vi "OCR test bench.vi"() -> ()   [LabVIEW 2017]
uses:
  <vilib>/vision/NI_Vision_Development_Module.lvlib
  <vilib>/userdefined/High Color/IMAQdx.ctl
  <vilib>/vision/Image Controls.llb/IMAQ Image.ctl
  <vilib>/vision/Avi.llb/IMAQ AVI2 Refnum.ctl
  Controls/Refnums.ctl
  Controls/Room Dimensions.ctl
  Controls/Dimensions.ctl
  Controls/Frame Grabber Data.ctl
  <vilib>/Utility/miscctls.llb/LVOutOfRangeActionTypeDef.ctl
  Controls/Crop Type.ctl
  Controls/Crop Video State.ctl
  <vilib>/vision/OCR.llb/IMAQ OCR Character Report 2.ctl
panel:
  out "Character Reports":T1[](array[typedef]) {"Character Statistics"."Threshold Range"."Upper value" format="%.2f"; "Character Statistics"."Threshold Range"."Lower value" format="%.2f"}
  in  "Range":cluster{"Lower value":sgl, "Upper value":sgl}={"Lower value"=128.0, "Upper value"=255.0} {"Upper value" format="%.2f"; "Lower value" format="%.2f"}
  out "Cropped":T2(plugin-control)
  in  "Stop Button":bool
  in  "Blue or Luminance":cluster{"Min":i32, "Max":i32}(slide)={"Min"=70, "Max"=183} scale=0.0..255.0
  in  "Green or Saturation":cluster{"Min":i32, "Max":i32}(slide)={"Min"=51, "Max"=206} scale=0.0..255.0
  in  "Red or Hue":cluster{"Min":i32, "Max":i32}(slide)={"Min"=217, "Max"=15} scale=0.0..255.0
  out "Thresh Image":T2(plugin-control)
  out "Frame":T2(plugin-control)
  out "Reference zero image":T2(plugin-control)
  in  "Frame Number":u32 max=30
  out "Read String":string
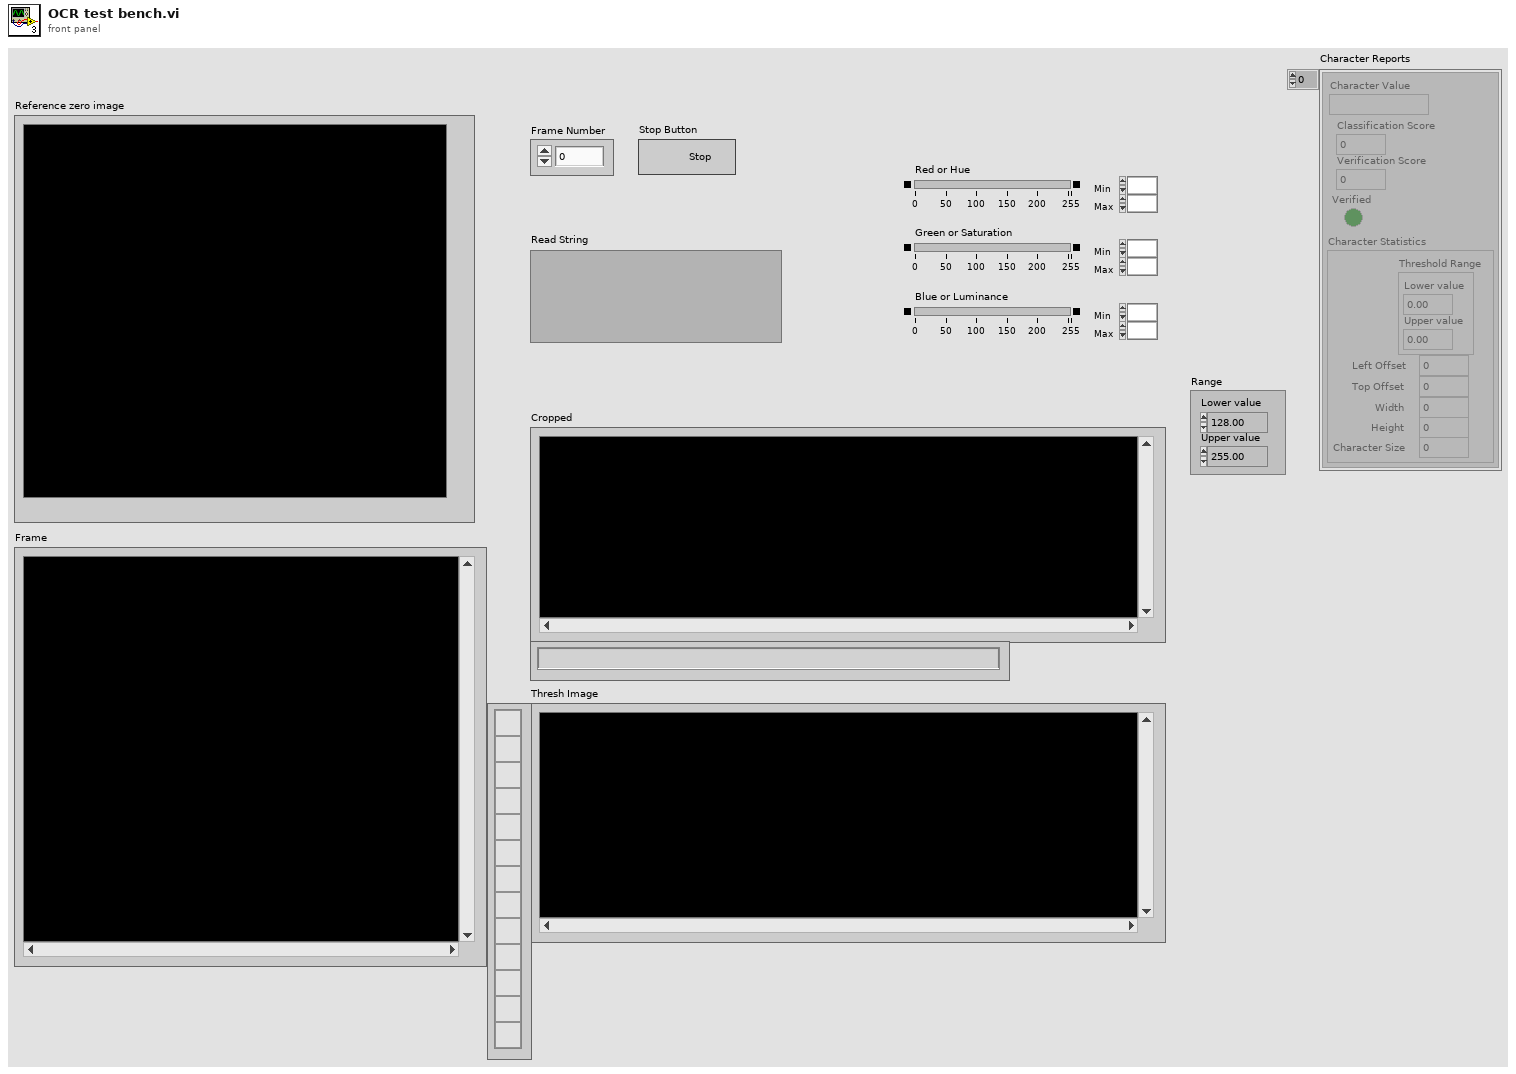
[diagram p1: front panel]
types:
  T1 = typedef "IMAQ OCR Character Report 2.ctl" = cluster{"Character Value":string, "Classification Score":i32, "Verification Score":i32, "Verified":bool, "Character Statistics":cluster{"Threshold Range":cluster{"Lower value":sgl, "Upper value":sgl}, "Left Offset":i32, "Top Offset":i32, "Width":i32, "Height":i32, "Character Size":i32}}
  T2 = typedef "IMAQ Image.ctl" = refnum<image>
  T3 = typedef "LVOutOfRangeActionTypeDef.ctl" = cluster{"Out of Range Action Minimum":u8, "Out of Range Action Maximum":u8, "Out of Range Action Increment":u8}
  T4 = typedef "Frame Grabber Data.ctl" = cluster{"Camera Session":T5, "Frame":T2, "AVI Refnum":T6, "Codecs":string[], "Frame number":u32, "Tracking File Refnum":refnum<file>, "Tick Count":u32, "Probe Object":refnum<vi>, "Playback Probe Data":dbl[][], "Total no frames playback":i32, "Video FPS":dbl, "Camera connected?":bool, "Scene":refnum<vi>, "Cropped Frame":T2, "Tracker FPS":dbl, "Crop ROI":i32[], "Presentation Values":string[], "Elapsed time (ms)":u32, "Camera frames playback":u32, "Refnums":T7, "Dimensions":T8, "Playback Data As Strings":string[][], "Cropped Tracking File Refnum":refnum<file>, "Cropped AVI Refnum":T6, "Header":string[], "Total euclidian distance":dbl, "Annotation File Path":path, "Playback File Path":path, "Size per frame":dbl, "Ground Truth File Refnum":refnum<file>, "Annotation Array":string[], "Annotation TIFFs Folder":path, "overwriting open file?":bool, "Image Sequence":T2[], "Video/Image Flag":T10, "Image sequence?":bool, "Image sequence filenames":string[], "Mask":T2, "Crop Type":T11}
  T5 = typedef "IMAQdx.ctl" = refnum<k21>
  T6 = typedef "IMAQ AVI2 Refnum.ctl" = refnum<k20>
  T7 = typedef "Refnums.ctl" = cluster{"Live Refnum":refnum<vi>, "Record Refnum":refnum<vi>, "Playback Refnum":refnum<vi>, "Frame Slider Refnum":refnum<vi>, "Pause Refnum":refnum<vi>, "Home Refnum":refnum<vi>, "Set Crop Refnum":refnum<vi>, "Clear Crop Refnum":refnum<vi>, "stop refnum":refnum<vi>, "Playback Rate Refnum":refnum<vi>, "Presentation Refnum":refnum<vi>, "Crop Time Frame Slider Refnum":refnum<vi>, "Cancel Save Refnum":refnum<vi>, "Reverse Playback Refnum":refnum<vi>, "Recording Settings Refnum":refnum<vi>, "Continuous Playback Refnum":refnum<vi>, "Annotation Refnum":refnum<vi>, "Export All Refnum":refnum<vi>, "Export List Refnum":refnum<vi>, "Fill List Refnum":refnum<vi>, "Save Crop Refnum":refnum<vi>, "Skip Forward Refnum":refnum<vi>, "Skip Backward Refnum":refnum<vi>, "Single Annotation Refnum":refnum<vi>, "Load Video Refnum":refnum<vi>, "Set Start Refnum":refnum<vi>, "Set End Refnum":refnum<vi>, "Add to List Refnum":refnum<vi>, "List of Annotations Refnum":refnum<vi>, "Camera Frame Refnum":refnum<vi>, "Load Image Refnum":refnum<vi>, "Saving Refnum":refnum<vi>}
  T8 = typedef "Dimensions.ctl" = cluster{"Probe Dimensions":cluster{"Probe Width":sgl, "Probe Depth":sgl, "Probe Height":sgl}, "Room Dimensions":T9}
  T9 = typedef "Room Dimensions.ctl" = cluster{"Room Width":dbl, "Room Depth":dbl, "Room Height":dbl}
  T10 = typedef "Crop Video State.ctl" = enum16{"Init", "Wait", "Load Image", "Load Video", "Play/Pause", "Playback Video Frame", "Display Image", "Save Image Sequence", "Save Video", "Export List", "Export All", "Close", "Set Crop Area", "Reset Crop Area", "Crop Inside", "Crop Outside", "Multi-Crop", "Re-Open Files", "Annotate Frame", "Annotate Clip", "Add to List", "Fill List", "Set Start", "Set End", "Error Handling", "Shutdown"}
  T11 = typedef "Crop Type.ctl" = enum16{"Rectangle", "Annulus"}
  T12 = cluster{"Global Rectangle":i32[], "Contours":cluster{"ID":enum32{"External", "Internal"}, "Type":u32, "Coordinates":i32[]}[]}
  T13 = typedef "Image Type" = u32
  T14 = typedef "IMAQ OCR Session.ctl" = refnum<k1>
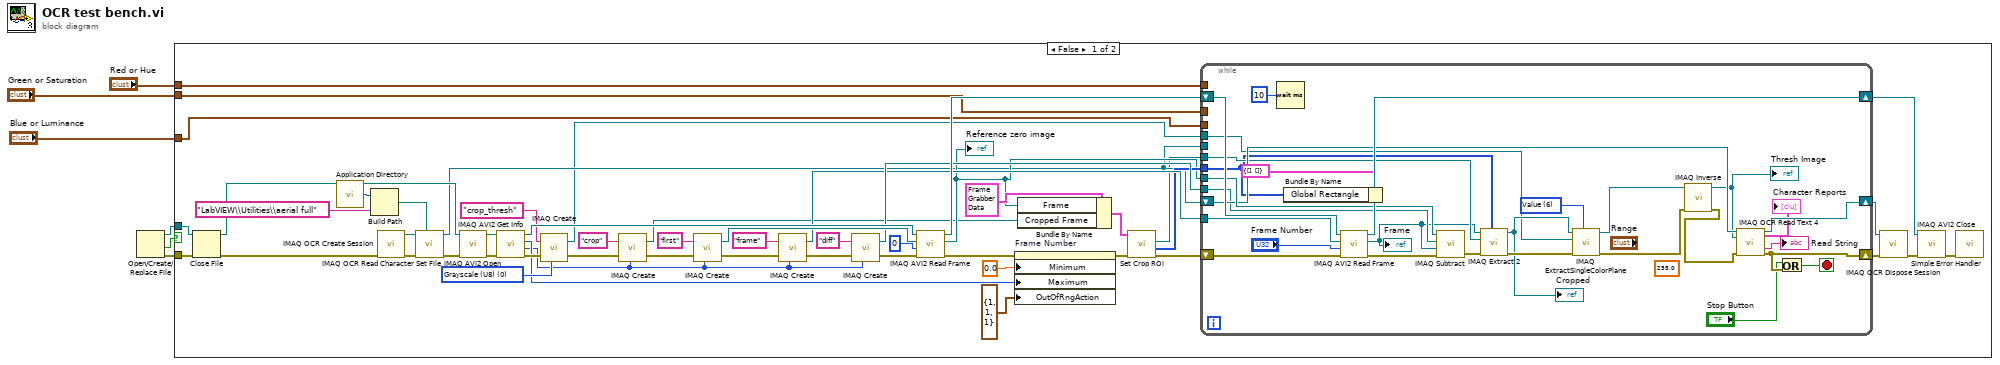
[diagram p0: block diagram]
diagram:
  n1 = Open/Create/Replace File() -> (refnum out=w6:refnum<file>, cancelled=w4:bool, error out=w5:errorcluster)  [unwired: 6 in]
  n2 = case shown="False" w4 {
    tunnel: w6 -> [w41 _]
    tunnel: w5 -> [w44 _]
    tunnel: "Red or Hue" -> [w17 _]
    tunnel: "Green or Saturation" -> [w16 _]
    tunnel: "Blue or Luminance" -> [w15 _]
    frame False {
      w14 = T13 0 items=["Grayscale (U8)", "Grayscale (I16)", "Grayscale (SGL)", "Complex (CSG)", "RGB (U32)", "HSL (U32)", "RGB (U64)", "Grayscale (U16)"] ("Image Type")
      n3 = Close File(refnum=w41, error in=w44) -> (path=w42:path, error out=w43:errorcluster)
      n4 = call <vilib>:"Application Directory.vi"() -> ("Application Directory"=w26:path)
      n5 = Build Path(base path=w26, name or relative path="LabVIEW\\Utilities\\aerial full") -> (appended path=w24:path)
      n6 = call "IMAQ OCR Create Session"("error in (no error)"=w43) -> ("error out"=w30:errorcluster, "IMAQ OCR Session"=w29:T14)  [unwired: 9 in]
      n7 = call "IMAQ OCR Read Character Set File"("File Path"=w24, "error in (no error)"=w30, "IMAQ OCR Session"=w29) -> ("error out"=w27:errorcluster, "IMAQ OCR Session (dup)"=w28:T14)  [unwired: 6 in, 1 out]
      n8 = call "IMAQ AVI2 Open"("error in (no error)"=w27, "AVI File Path"=w42) -> ("error out"=w58:errorcluster, "AVI Refnum"=w59:T6)  [unwired: 8 in]
      n9 = call "IMAQ AVI2 Get Info"("error in (no error)"=w58, "AVI Refnum"=w59) -> ("error out"=w21:errorcluster, "Image Type"=w9:T13, "Number of Frames"=w10:u32, "AVI Refnum (duplicate)"=w57:T6)  [unwired: 5 in, 1 out]
      n10 = call "IMAQ Create"("Image Name"="crop_thresh", "Image Type"=w14, "error in (no error)"=w21) -> ("New Image"=w18:T2, "error out"=w20:errorcluster)  [unwired: 2 in]
      n11 = call "IMAQ Create"("Image Name"="crop", "Image Type"=w9, "error in (no error)"=w20) -> ("New Image"=w23:T2, "error out"=w32:errorcluster)  [unwired: 2 in]
      n12 = call "IMAQ Create"("Image Name"="first", "Image Type"=w9, "error in (no error)"=w32) -> ("New Image"=w53:T2, "error out"=w54:errorcluster)  [unwired: 2 in]
      n13 = call "IMAQ Create"("Image Name"="frame", "Image Type"=w9, "error in (no error)"=w54) -> ("New Image"=w45:T2, "error out"=w50:errorcluster)  [unwired: 2 in]
      n14 = call "IMAQ Create"("Image Name"="diff", "Image Type"=w9, "error in (no error)"=w50) -> ("New Image"=w48:T2, "error out"=w49:errorcluster)  [unwired: 2 in]
      n15 = call "IMAQ AVI2 Read Frame"("error in (no error)"=w49, "Frame Number"=u32 0, "Image"=w53, "AVI Refnum"=w57) -> ("error out"=w8:errorcluster, "Image Out"=w31:T2, "AVI Refnum (duplicate)"=w52:T6)  [unwired: 5 in]
      "Reference zero image" <- w31
      n16 = property on="Frame Number" class="DigNum (strict)"(error in=w8, "Minimum"=0.0 ("Data Entry Limits:Minimum"), "Maximum"=w10, "OutOfRngAction"=T3 {"Out of Range Action Minimum"=1, "Out of Range Action Maximum"=1, "Out of Range Action Increment"=1} ("Response to Value Outside Limits")) -> (error out=w7:errorcluster)  [unwired: 1 in, 1 out]
      n17 = Bundle By Name(cluster=T4 {"Camera Session"="", "Frame"=refnum, "AVI Refnum"=refnum, "Codecs"=[], "Frame number"=0, "Tracking File Refnum"=refnum, "Tick Count"=0, "Probe Object"=refnum, "Playback Probe Data"=[], "Total no frames playback"=0, "Video FPS"=0.0, "Camera connected?"=FALSE, "Scene"=refnum, "Cropped Frame"=refnum, "Tracker FPS"=0.0, "Crop ROI"=[], "Presentation Values"=[], "Elapsed time (ms)"=0, "Camera frames playback"=0, "Refnums"={"Live Refnum"=refnum, "Record Refnum"=refnum, "Playback Refnum"=refnum, "Frame Slider Refnum"=refnum, "Pause Refnum"=refnum, "Home Refnum"=refnum, "Set Crop Refnum"=refnum, "Clear Crop Refnum"=refnum, "stop refnum"=refnum, "Playback Rate Refnum"=refnum, "Presentation Refnum"=refnum, "Crop Time Frame Slider Refnum"=refnum, "Cancel Save Refnum"=refnum, "Reverse Playback Refnum"=refnum, "Recording Settings Refnum"=refnum, "Continuous Playback Refnum"=refnum, "Annotation Refnum"=refnum, "Export All Refnum"=refnum, "Export List Refnum"=refnum, "Fill List Refnum"=refnum, "Save Crop Refnum"=refnum, "Skip Forward Refnum"=refnum, "Skip Backward Refnum"=refnum, "Single Annotation Refnum"=refnum, "Load Video Refnum"=refnum, "Set Start Refnum"=refnum, "Set End Refnum"=refnum, "Add to List Refnum"=refnum, "List of Annotations Refnum"=refnum, "Camera Frame Refnum"=refnum, "Load Image Refnum"=refnum, "Saving Refnum"=refnum}, "Dimensions"={"Probe Dimensions"={"Probe Width"=0.0, "Probe Depth"=0.0, "Probe Height"=0.0}, "Room Dimensions"={"Room Width"=0.0, "Room Depth"=0.0, "Room Height"=0.0}}, "Playback Data As Strings"=[], "Cropped Tracking File Refnum"=refnum, "Cropped AVI Refnum"=refnum, "Header"=[], "Total euclidian distance"=0.0, "Annotation File Path"=path "", "Playback File Path"=path "", "Size per frame"=0.0, "Ground Truth File Refnum"=refnum, "Annotation Array"=[], "Annotation TIFFs Folder"=path "", "overwriting open file?"=FALSE, "Image Sequence"=[], "Video/Image Flag"=enum."Init", "Image sequence?"=FALSE, "Image sequence filenames"=[], "Mask"=refnum, "Crop Type"=enum."Rectangle"} ("Frame Grabber Data in"), "Frame"=w31, "Cropped Frame"=w23) -> (w34:T4)
      n18 = call "Set Crop ROI.vi"("error in (no error)"=w7, "Frame Grabber Data in"=w34) -> ("error out"=w36:errorcluster, "Crop ROI"=w37:i32[], "Image Out"=w22:T2)  [unwired: 4 in, 3 out]
      n19 = while {
        shift-right: [w73] -> w47
        shift-left: w36 -> [w88]
        tunnel: w45 -> [w87]
        shift-right: [w85] -> w39
        shift-left: w52 -> [w86]
        tunnel: w31 -> [w83]
        tunnel: w48 -> [w79]
        tunnel: w28 -> [_]
        shift-right: [w82] -> w46
        shift-left: w28 -> [w81]
        tunnel: w37 -> [w75]
        tunnel: w22 -> [w76]
        tunnel: w18 -> [w61]
        tunnel: w17 -> [_]
        tunnel: w16 -> [_]
        tunnel: w15 -> [_]
        stop <- w72 stop-if-true
        (unwired) sgl 255.0 ("Replace Value")
        w68 = 6 items=["Red", "Green", "Blue", "Hue", "Saturation", "Luminance", "Value", "Intensity"] ("Color Plane")
        n20 = Wait (ms)(milliseconds to wait=u32 10) -> ()  [unwired: 1 out]
        n21 = Bundle By Name(cluster=T12 {"Global Rectangle"=[], "Contours"=[]} ("ROI Descriptor"), "Global Rectangle"=w75) -> ()  [unwired: 1 out]
        n22 = call "IMAQ AVI2 Read Frame"("error in (no error)"=w88, "Frame Number"="Frame Number", "Image"=w87, "AVI Refnum"=w86) -> ("error out"=w84:errorcluster, "Image Out"=w67:T2, "AVI Refnum (duplicate)"=w85:T6)  [unwired: 5 in]
        "Frame" <- w67
        n23 = call "IMAQ Subtract"("Image Src A"=w83, "Image Dst"=w79, "Image Src B"=w67, "error in (no error)"=w84) -> ("error out"=w70:errorcluster)  [unwired: 3 in, 1 out]
        n24 = call "IMAQ Extract 2"("Optional Rectangle"=w75, "error in (no error)"=w70, "Image Dst"=w76, "Image Src"=w67) -> ("error out"=w69:errorcluster, "Image Dst Out"=w63:T2)  [unwired: 6 in]
        "Cropped" <- w63
        n25 = call "IMAQ ExtractSingleColorPlane"("Color Plane"=w68, "error in (no error)"=w69, "Image Dst"=w61, "Image Src"=w63) -> ("error out"=w66:errorcluster, "Image Dst Out"=w62:T2)  [unwired: 6 in]
        n26 = call "IMAQ Inverse"("error in (no error)"=w66, "Image Src"=w62) -> ("error out"=w65:errorcluster, "Image Dst Out"=w64:T2)  [unwired: 8 in]
        "Thresh Image" <- w64
        n27 = call "IMAQ OCR Read Text 4"("IMAQ OCR Session"=w81, "Image"=w64, "error in (no error)"=w65) -> ("Character Reports"=→"Character Reports":T1[], "IMAQ OCR Session (dup)"=w82:T14, "Read String"=→"Read String":string, "error out"=w73:errorcluster)  [unwired: 6 in, 3 out]
        n28 = Or(x="Stop Button", y=w73) -> (x .or. y?=w72:bool)
      }
      n29 = call "IMAQ OCR Dispose Session"("error in (no error)"=w47, "IMAQ OCR Session"=w46) -> ("error out"=w40:errorcluster)  [unwired: 9 in]
      n30 = call "IMAQ AVI2 Close"("error in (no error)"=w40, "AVI Refnum"=w39) -> ("error out"=w38:errorcluster)  [unwired: 9 in]
      n31 = call <vilib>:"Simple Error Handler.vi"("error in (no error)"=w38) -> ()  [unwired: 4 in, 5 out]
    }
    frame True {
    }
  }
